vi "Wait For Acquisition.vi"(8 "error in (no error)":errorcluster) -> (0 "error out":errorcluster, 3 "function return":u32)   [LabVIEW 2014, in "atmcd32d.lvlib"]
doc: "unsigned int WINAPI WaitForAcquisition(void);"
uses:
  atmcd32d.lvlib
  atmcd32d.dll
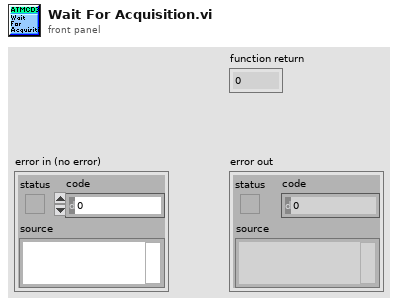
[diagram p1: front panel]
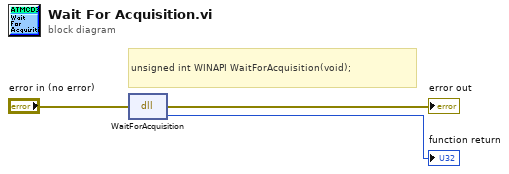
[diagram p0: block diagram]
diagram:
  # "unsigned int WINAPI WaitForAcquisition(void);"
  n1 = dll-call lib="C:/Users/Bakir/Documents/Lambda2-Testing/lib/Andorlib/atmcd32d.*" fn="WaitForAcquisition"(error in="error in (no error)") -> (error out=→"error out":errorcluster, →"function return":u32)  [unwired: 2 in, 1 out]
